vi "Read String.vi"(8 "error in (no error)":errorcluster, 11 "Bus in":refnum<class "Bus.lvclass">) -> (0 "error out":errorcluster, 1 "Bytes Read":i32, 2 "String Read":string, 3 "Bus out":refnum<class "Bus.lvclass">)   [LabVIEW 2024, in "Bus.lvclass"]
doc: "Bus.lvclass:Read String.vi\n\nThis is the template for the Read String VI forthe Bus class.\n\nInstrument Communication Module Version 1.0\nJuly, 2017 Original Code Consulting David Thomson\n www.originalcode.com"
uses:
  Bus.lvclass
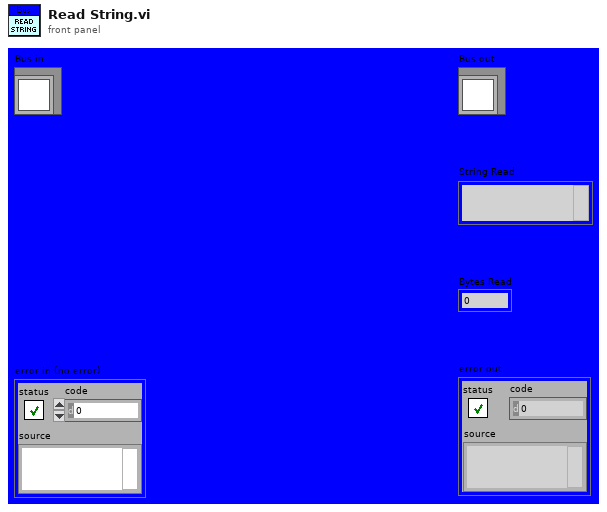
[diagram p1: front panel]
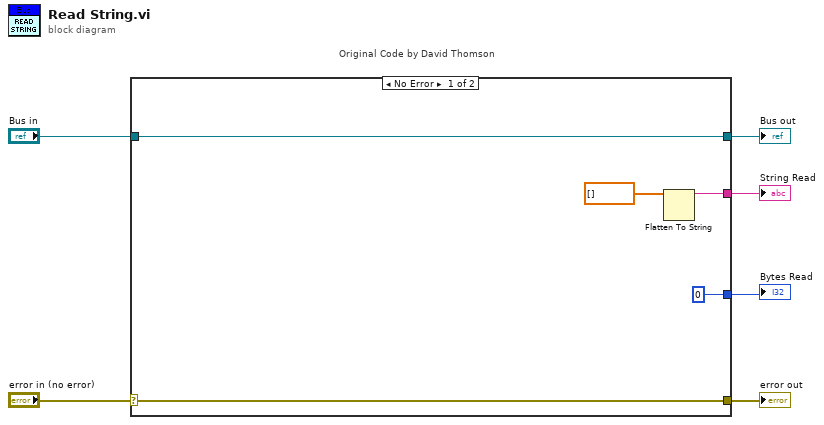
[diagram p0: block diagram]
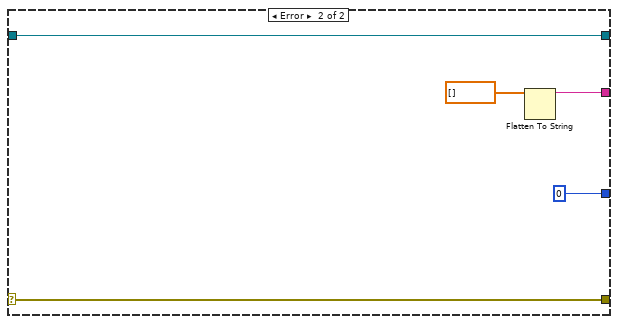
[diagram p2: hidden frame]
diagram:
  n1 = case "Original Code by David Thomson" shown="No Error" "error in (no error)" {
    selector: "error in (no error)" -> [w10 w16]
    tunnel: [w10 w16] -> w5
    tunnel: [w11 w15] -> w3
    tunnel: "Bus in" -> [w11 w15]
    tunnel: [w9 w13] -> w2
    tunnel: [0 ("Bytes Read") 0 ("Bytes Read")] -> w1
    frame No Error {
      n2 = Flatten To String(anything=dbl[] []) -> (data string=w9:string)  [unwired: 3 in, 2 out]
    }
    frame Error {
      n3 = Flatten To String(anything=dbl[] []) -> (data string=w13:string)  [unwired: 3 in, 2 out]
    }
  }
  "error out" <- w5
  "Bus out" <- w3
  "String Read" <- w2
  "Bytes Read" <- w1
